vi "Wait Until Canceled.vi"(8 "error in (no error)":errorcluster, 9 "polling interval (ms)":i32=10, 10 "measurement complete":refnum<user-event>, 11 "MeasurementContext in":refnum<class "Measure Call Context.lvclass">) -> (0 "error out":errorcluster, 2 "is canceled?":bool, 3 "MeasurementContext out":refnum<class "Measure Call Context.lvclass">)   [LabVIEW 2020, in "Keysight 34401A DMM Measurement.lvlib"]
uses:
  Keysight 34401A DMM Measurement.lvlib
  <vilib>/Plug-In SDKs/Measurements/Measure Call Context/Measure Call Context.lvclass
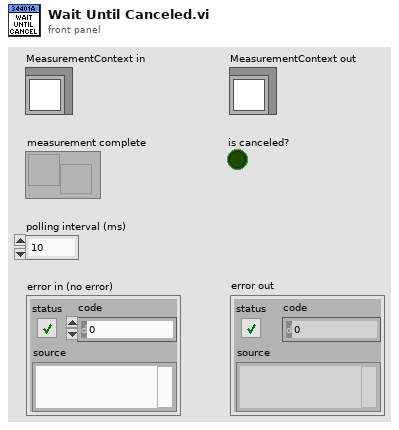
[diagram p1: front panel]
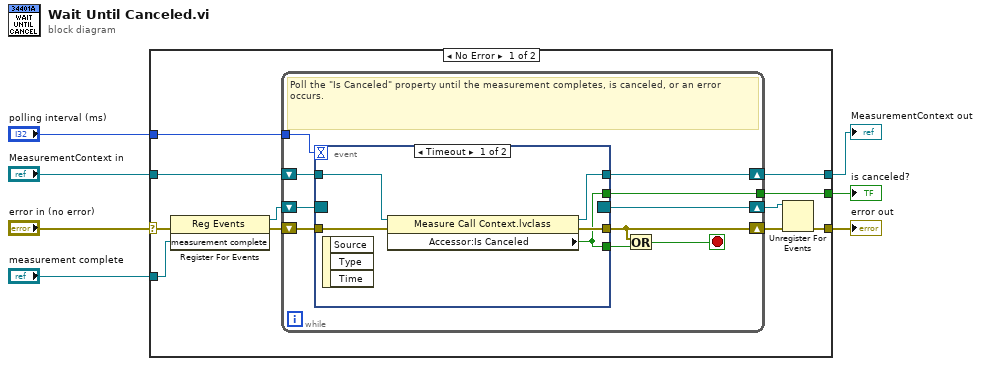
[diagram p0: block diagram]
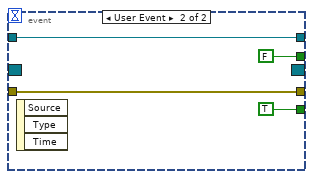
[diagram p2: hidden frame]
diagram:
  n1 = case shown="No Error" "error in (no error)" {
    selector: "error in (no error)" -> [w8 w39]
    tunnel: "MeasurementContext in" -> [w18 w38]
    tunnel: [w17 w38] -> w6
    tunnel: [w16 _] -> w5
    tunnel: "polling interval (ms)" -> [w15 _]
    tunnel: "measurement complete" -> [w14 _]
    tunnel: [w9 w39] -> w2
    frame No Error {
      n2 = register-events(error in=w8, w14) -> (reference out=w13:refnum<event-registration>, error out=w12:errorcluster)  [unwired: 1 in]
      n3 = while {
        shift-right: [w24] -> w10
        shift-left: w12 -> [w27]
        shift-right: [w26] -> w17
        shift-left: w18 -> [w28]
        tunnel: [w21] -> w16
        tunnel: w15 -> [w22]
        shift-right: [w19] -> w11
        shift-left: w13 -> [w20]
        stop <- w25 stop-if-true
        # "Poll the \"Is Canceled\" property until the measurement completes, is canceled, or an error occurs."
        n4 = event shown="[0] Timeout" {
          selector: w20 -> [_ _]
          dyn-events: [_ _] -> w19
          timeout: w22 -> [_ _]
          tunnel: w28 -> [w33 w35]
          tunnel: w27 -> [w32 w34]
          tunnel: [w31 w35] -> w26
          tunnel: [w30 w34] -> w24
          tunnel: [w29 TRUE ("Accessor:Is Canceled")] -> w23
          tunnel: [w29 FALSE ("Accessor:Is Canceled")] -> w21
          event Timeout {
            n5 = event-data() -> ()  [unwired: 1 in, 3 out]
            n6 = property class="Measure Call Context.lvclass"(reference=w33, error in=w32) -> (reference out=w31:refnum<class "Measure Call Context.lvclass">, error out=w30:errorcluster, "Accessor:Is Canceled"=w29:bool)
          }
          event User Event {
            n7 = event-data() -> ()  [unwired: 1 in, 3 out]
          }
        }
        n8 = Or(x=w24, y=w23) -> (x .or. y?=w25:bool)
      }
      n9 = Unregister For Events(event registration refnum=w11, error in=w10) -> (error out=w9:errorcluster)
    }
    frame Error {
    }
  }
  "error out" <- w2
  "MeasurementContext out" <- w6
  "is canceled?" <- w5
